vi "Start.vi"(8 "error in (no error)":errorcluster, 9 "Channel Data (DBLs Only)":T1={"Inputs"={"Data to Server"=1.0}, "Outputs"={"Data from Server"=0.0}}, 10 "Real-Time System Data":T2, 11 "Configuration Data":T3={"Timeout (ms)"=100, "Server IP"="localhost", "Port"=6340}) -> (0 "error out":errorcluster, 1 "Channel Data (DBLs Only)":T1={"Inputs"={"Data to Server"=1.0}, "Outputs"={"Data from Server"=0.0}}, 2 "Real-Time System Data":T2, 3 "Configuration Data":T3={"Timeout (ms)"=100, "Server IP"="localhost", "Port"=6340})   [LabVIEW 2013, in "TCPIP Custom Device.lvlib"]
uses:
  TCPIP Custom Device.lvlib
  Configuration Data.ctl
  Real-Time System Data.ctl
  Channel Data.ctl
panel:
  # "Controls"
  # "Indicators"
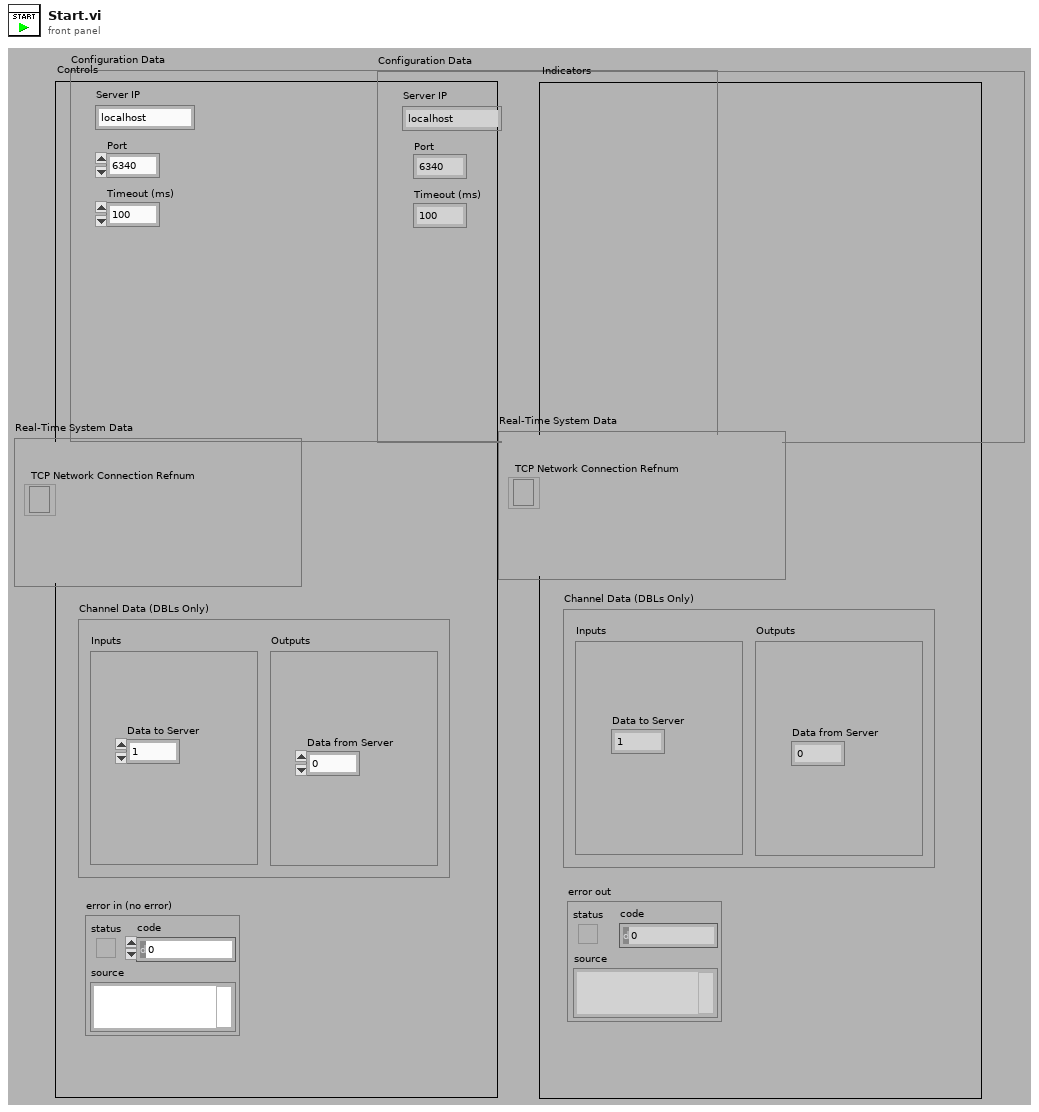
[diagram p1: front panel]
types:
  T1 = typedef "TCPIP Custom Device.lvlib/Channel Data.ctl" = cluster{"Inputs":cluster{"Data to Server":dbl}, "Outputs":cluster{"Data from Server":dbl}}
  T2 = typedef "TCPIP Custom Device.lvlib/Real-Time System Data.ctl" = cluster{"TCP Network Connection Refnum":refnum<k5>}
  T3 = typedef "TCPIP Custom Device.lvlib/Configuration Data.ctl" = cluster{"Timeout (ms)":i32, "Server IP":string, "Port":i32}
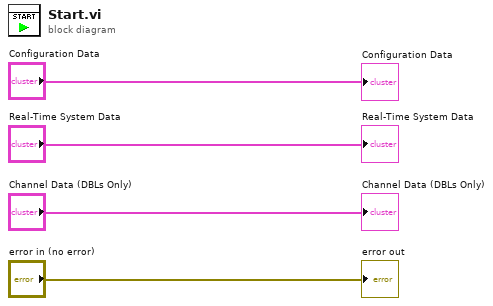
[diagram p0: block diagram]
diagram:
  "error out" <- "error in (no error)"
  "Configuration Data" <- "Configuration Data"
  "Real-Time System Data" <- "Real-Time System Data"
  "Channel Data (DBLs Only)" <- "Channel Data (DBLs Only)"
